vi "Publish Data.vi"(6 "Publish Time (Use Current Time)":timestamp, 8 "error in (no error)":errorcluster, 9 "Data to Publish":variant, 10 "Datum Name":string, 11 "IModel in":refnum<class "IModel.lvclass">) -> (0 "error out":errorcluster, 3 "IModel out":refnum<class "IModel.lvclass">)   [LabVIEW 2019, in "IModel.lvlib" / "IModel.lvclass"]
uses:
  <vilib>/gpm_packages/@cs/mva-core/Source/IModel/IModel/IModel.lvclass
  C:/Program Files/National Instruments/LabVIEW 2019/vi.lib/gpm_packages/@cs/mva-core/Source/IObserver/IObserver/IObserver.lvclass
  <vilib>/gpm_packages/@cs/mva-core/Source/IObserver/IObserver/IObserver.lvclass/IObserver.ctl
  <vilib>/gpm_packages/@cs/mva-core/Source/IModel/IModel/IModel.lvclass/IModel.ctl
  <vilib>/gpm_packages/@cs/mva-core/Source/IMediator/PublishRequest/PublishRequest.lvclass
  <vilib>/gpm_packages/@cs/mva-core/Source/IMediator/PublishRequest/PublishRequest.lvclass/PublishRequest.ctl
  <vilib>/gpm_packages/@cs/mva-core/Source/IMediator/IMediator Messages/Publish Msg/Publish Msg.lvclass/Publish Msg.ctl
  <vilib>/gpm_packages/@cs/actor-framework-messages/Source/RoundTripMessage/RoundTripMessage.lvclass/RoundTripMessage.ctl
  <vilib>/ActorFramework/Message Enqueuer/Message Enqueuer.lvclass/Message Enqueuer.ctl
  <vilib>/gpm_packages/@cs/actor-framework-messages/Source/RoundTripMessage/Return Round-Trip Message.vi
  <vilib>/ActorFramework/Message Enqueuer/Enqueue.vi
  <vilib>/gpm_packages/@cs/mva-core/Source/IMediator/IMediator Messages/Publish Msg/Publish Msg.lvclass
  C:/Program Files/National Instruments/LabVIEW 2019/vi.lib/gpm_packages/@cs/actor-framework-messages/Source/RoundTripMessage/RoundTripMessage.lvclass
  <vilib>/gpm_packages/@cs/actor-framework-messages/Source/RoundTripMessage/RoundTripMessage.lvclass
  C:/Program Files/National Instruments/LabVIEW 2019/vi.lib/ActorFramework/Message/Message.lvclass
  <vilib>/Utility/error.llb/Error Cluster From Error Code.vi
  <vilib>/ActorFramework/Message Priority Queue/Priority Enqueue.vi
  <vilib>/gpm_packages/@cs/mva-core/Source/IObserver/IObserver/IObserver.lvclass
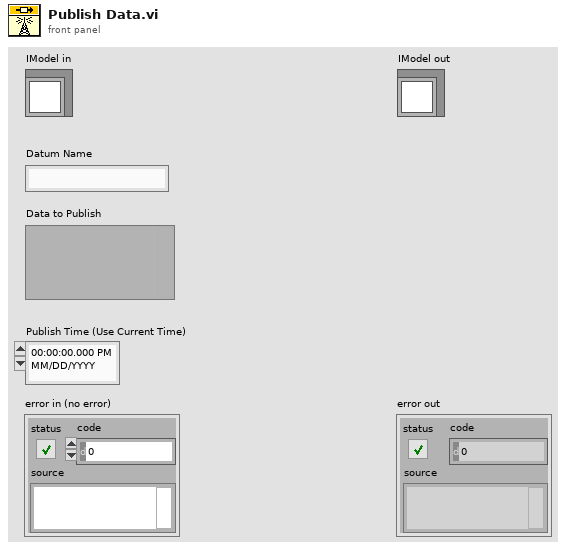
[diagram p1: front panel]
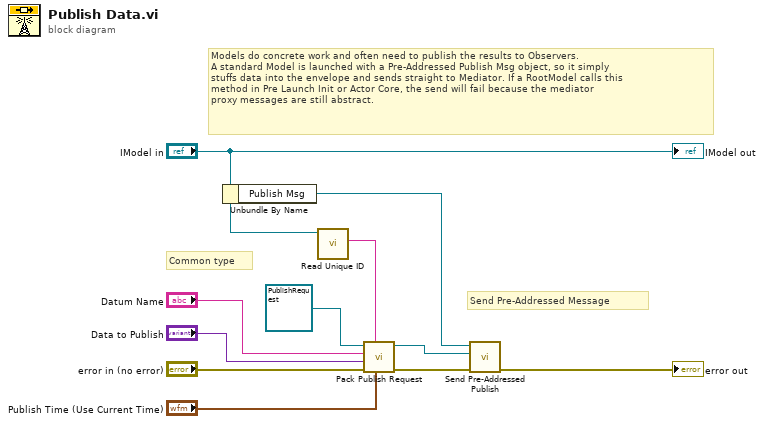
[diagram p0: block diagram]
diagram:
  # "Common type"
  # "Models do concrete work and often need to publish the results to Observers.\nA standard Model is launched with a Pre-Addressed Publish Msg object, so it simply\nstuffs data into the envelope and sends straight to Mediator. If a RootModel calls this\nmethod in Pre Launch Init or Actor Core, the send will fail because the mediator\nproxy messages are still abstract."
  # "Send Pre-Addressed Message"
  n1 = Unbundle By Name("IModel in") -> ("Publish Msg"=w11:refnum<class "Publish Msg.lvclass">)
  n2 = call <vilib>:"Read Unique ID.vi"("IObserver In"="IModel in") -> ("Unique ID"=w4:string)  [unwired: 10 in]
  n3 = call <vilib>:"Pack Publish Request.vi"("Publication Time (Use Current Time)"="Publish Time (Use Current Time)", "Publisher ID"=w4, "error in (no error)"="error in (no error)", "Value"="Data to Publish", "Datum Name"="Datum Name", "PublishRequest In"=refnum<class "PublishRequest.lvclass"> refnum ("IMediator.lvlib:PublishRequest.lvclass")) -> ("error out"=w2:errorcluster, "PublishRequest Out"=w5:refnum<class "PublishRequest.lvclass">)  [unwired: 4 in]
  n4 = call <vilib>:"Send Pre-Addressed Publish.vi"("error in (no error)"=w2, "PublishRequest"=w5, "Publish Message"=w11) -> ("error out"=→"error out":errorcluster)  [unwired: 8 in]
  "IModel out" <- "IModel in"
